vi "Set_Source.vi"(6 "Source Status":T7, 7 "Establish Exp Conditions":bool, 8 "Traverse line":T3 {"Carrier_2 Q (l/min)" format="%#.2f"; "Row Duration (mins)" format="%#.1f"; "Row No" min=0; "Trace Gas Concentration (%)" min=0.0 format="%#_4f"; "Carrier_1 Q (l/min)" format="%#.2f"; "Tunnel Speed" format="%#.2f"; "Start X" format="%#.2f"; "Start Y" format="%#.2f"; "Start Z" format="%#.2f"; "End X" format="%#.2f"; "End Y" format="%#.2f"; "End Z" format="%#.2f"; "Averaging time (min)" min=0.0 format="%#.2f"}, 9 "Simulate/Run":T6) -> (0 "Status Cluster":T1, 1 "Flowrates (kg/min)":dbl[](array[numeric]) format="%.2f", 2 "Time Source Started":dbl, 3 "Flowrates Achieved?":bool, 4 "Source requested?":bool, 5 "Source Est Time":dbl format="%.2f")   [LabVIEW 2016]
uses:
  ADAM Client/Sub VIs/ADAM Controls/Client_Source_Status.ctl
  Controls/User_Specific_mode.ctl
  Traverse_cluster.ctl
  Spacing.ctl
  Controls/Multi_run_mode.ctl
  Status_Cluster.ctl
  Multi_Run_Status.ctl
  Globals/Trav_pos_global.vi
  Globals/Extra_Commands_Global.vi
panel:
  # "X           Y            Z"
  # "Start"
  # "End"
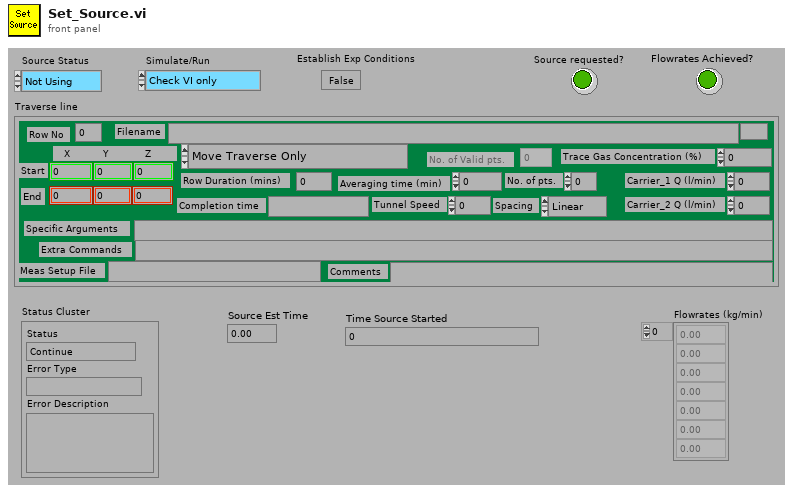
[diagram p1: front panel]
types:
  T1 = typedef "Status_Cluster.ctl" = cluster{"Status":T2, "Error Type":string, "Error Description":string}
  T2 = typedef "Multi_Run_Status.ctl" = enum16{"Continue", "Jump to Next Point", "Jump to Next Row", "Jump To Fall Back", "Terminate Run"}
  T3 = typedef "Traverse_cluster.ctl" = cluster{"Start X":sgl, "Start Y":sgl, "Start Z":sgl, "End X":sgl, "End Y":sgl, "End Z":sgl, "No. of pts.":i32, "Spacing":T4, "Filename":path, "Tunnel Speed":dbl, "Averaging time (min)":dbl, "Extra Commands":string, "Carrier_1 Q (l/min)":dbl, "Carrier_2 Q (l/min)":dbl, "Trace Gas Concentration (%)":dbl, "Specific Arguments":string, "Comments":string, "Row No":i32, "Row Type Selector":T5, "Completion time":string, "Row Duration (mins)":dbl, "No. of Valid pts.":i32, "Meas Setup File":string}
  T4 = typedef "Spacing.ctl" = enum16{"Linear", "Log", "Gauss", "Specified", "N/A"}
  T5 = typedef "Multi_run_mode.ctl" = enum16{"Move Traverse Only", "Set Tunnel Speed Only", "Set Source Only", "Set Measurement Conditions", "Single Measurement", "Vertical Profile", "Lateral Profile", "Longitudinal Profile", "Explore Volume", "Multi-Axis Profile", "Auto Calibrate", "Meas Fast FID Bkgnd", "Check Beam Power", "Scanning Valve Measurement", "Run VI Named:", "Set ADAM Ch", "Wait (minutes)", "Send Message", "Synchronize With:", "Fall Back to this Row", "Turn Off Row Repeating", "Blank Row", "Traverse 3D Volume"}
  T6 = typedef "User_Specific_mode.ctl" = enum16{"Check VI only", "Run VI"}
  T7 = typedef "Client_Source_Status.ctl" = enum16{"Not Using", "Using", "Must Have"}
  T8 = cluster{"Carrier_1 Q (l/min)":dbl, "Carrier_2 Q (l/min)":dbl, "Trace Gas Concentration (%)":dbl}
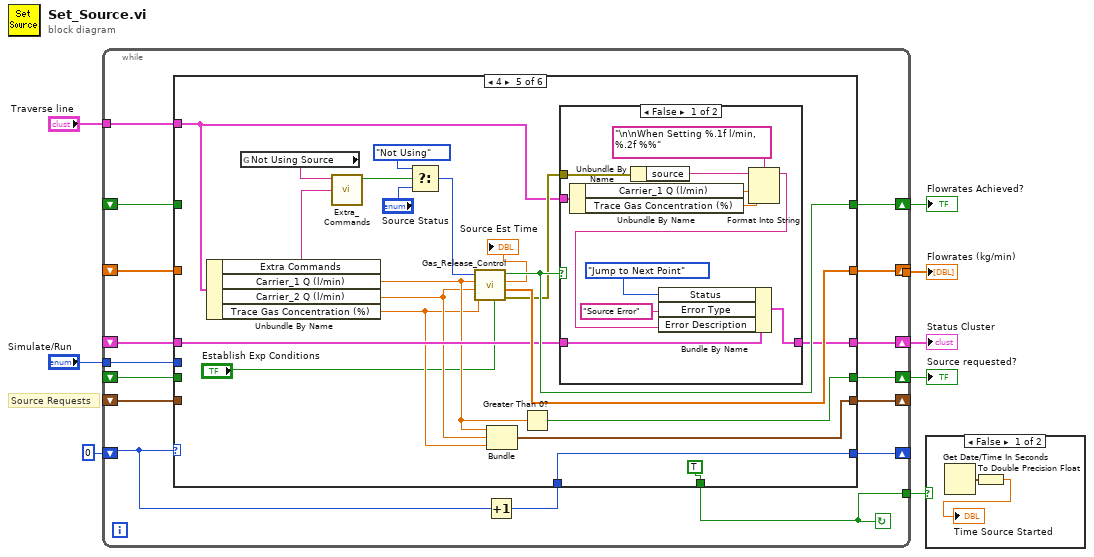
[diagram p0: block diagram]
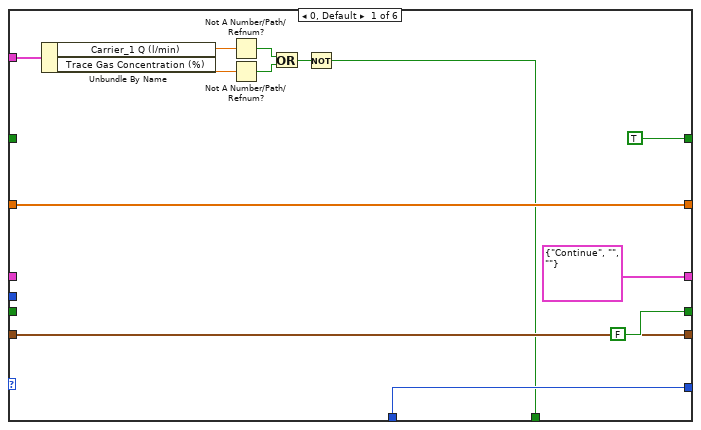
[diagram p3: hidden frame]
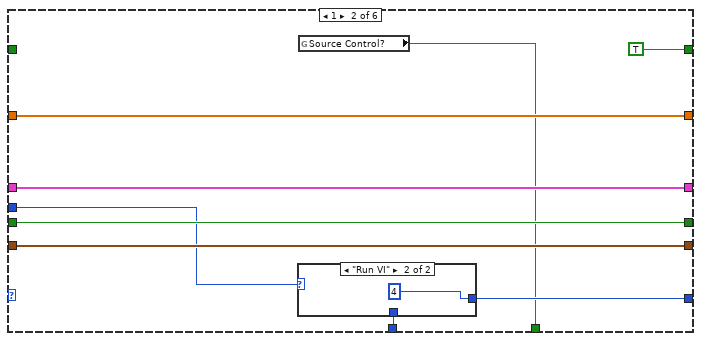
[diagram p4: hidden frame]
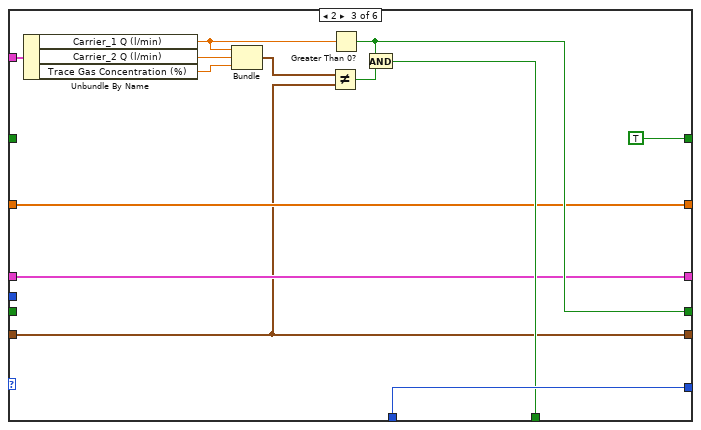
[diagram p6: hidden frame]
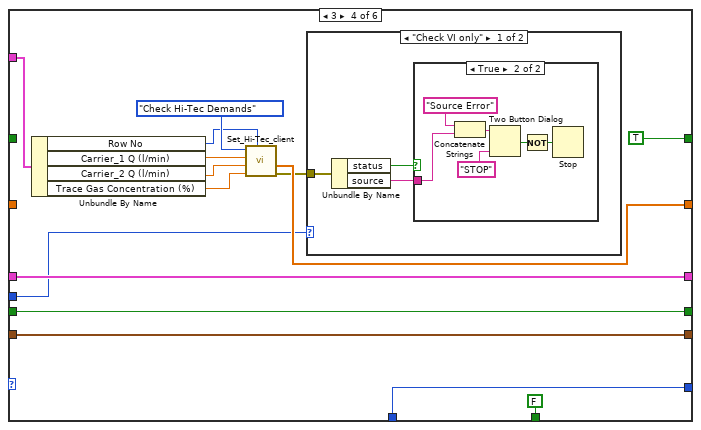
[diagram p7: hidden frame]
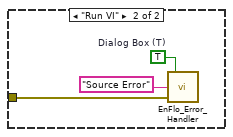
[diagram p9: hidden frame]
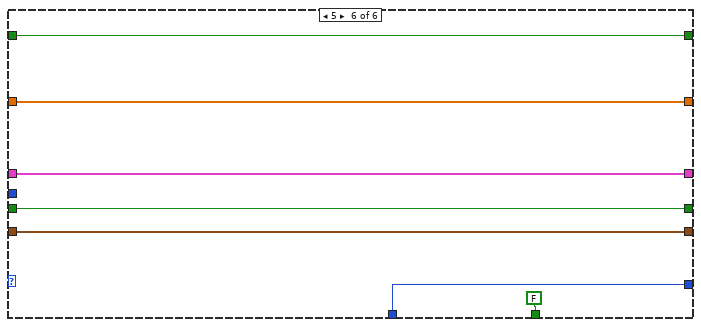
[diagram p11: hidden frame]
diagram:
  # "Source Requests"
  n1 = while {
    shift-left: _ -> [w12]
    shift-right: [w13] -> w4
    shift-left: _ -> [w14]
    shift-right: [w15] -> w5
    shift-left: _ -> [w16]
    shift-right: [w19] -> w6
    shift-left: 0 -> [w18]
    shift-right: [w20] -> _
    shift-left: _ -> [w21]
    shift-right: [w22] -> _
    tunnel: [w22] -> w8
    shift-left: _ -> [w24]
    shift-right: [w23] -> _
    tunnel: "Simulate/Run" -> [w11]
    tunnel: "Traverse line" -> [w10]
    tunnel: [w9] -> w1
    stop <- w9 continue-if-true
    n2 = Increment(x=w18) -> (x+1=w17:i32)
    n3 = case shown="4" w18 {
      tunnel: [w35 w46 w52 w71 w102 w123] -> w22
      tunnel: w24 -> [w32 w44 w50 w68 _ w127]
      tunnel: [w32 w44 w50 w68 w93 w127] -> w23
      tunnel: w21 -> [w35 w46 w52 _ _ w123]
      tunnel: [FALSE w40 w61 w69 w109 w128] -> w19
      tunnel: [TRUE ("Flowrates Achieved?") TRUE ("Flowrates Achieved?") TRUE ("Flowrates Achieved?") TRUE ("Flowrates Achieved?") w103 w122] -> w13
      tunnel: [w25 w38 w55 FALSE TRUE FALSE] -> w9
      tunnel: [w31 w43 w56 w67 w100 w126] -> w20
      tunnel: w17 -> [w31 w41 w56 w67 w100 w126]
      tunnel: w16 -> [_ w40 _ w69 _ w128]
      tunnel: [T1 {"Status"=enum."Continue", "Error Type"="", "Error Description"=""} ("Status Cluster") w42 w51 w65 w101 w124] -> w15
      tunnel: w14 -> [_ w42 w51 w65 w97 w124]
      tunnel: w12 -> [_ _ _ _ _ w122]
      tunnel: w11 -> [_ w39 _ w63 _ _]
      tunnel: w10 -> [w29 _ w49 w62 w91 _]
      frame 0, Default {
        n4 = Unbundle By Name(w29) -> ("Carrier_1 Q (l/min)"=w37:dbl, "Trace Gas Concentration (%)"=w30:dbl)
        n5 = Not A Number/Path/Refnum?(number/path/refnum=w37) -> (NaN/Path/Refnum?=w27:bool)
        n6 = Not A Number/Path/Refnum?(number/path/refnum=w30) -> (NaN/Path/Refnum?=w28:bool)
        n7 = Or(x=w27, y=w28) -> (x .or. y?=w26:bool)
        n8 = Not(x=w26) -> (.not. x?=w25:bool)
      }
      frame 1 {
        n9 = case shown="\"Run VI\"" w39 {
          tunnel: [w47 4] -> w43
          tunnel: w41 -> [w47 _]
          frame "Check VI only" {
          }
          frame "Run VI" {
          }
        }
        n10 = global read "Trav_pos_global.vi" "Source Control?"() -> (w38:bool)
      }
      frame 2 {
        n11 = Unbundle By Name(w49) -> ("Carrier_1 Q (l/min)"=w58:dbl, "Carrier_2 Q (l/min)"=w60:dbl, "Trace Gas Concentration (%)"=w59:dbl)
        n12 = Bundle("Carrier_1 Q (l/min)"=w58, "Carrier_2 Q (l/min)"=w60, "Trace Gas Concentration (%)"=w59) -> (w54:T8)  [unwired: 1 out]
        n13 = Not Equal?(x=w54, y=w50) -> (x != y?=w57:bool)
        n14 = Greater Than 0?(x=w58) -> (x > 0?=w61:bool)
        n15 = And(x=w61, y=w57) -> (x .and. y?=w55:bool)
      }
      frame 3 {
        n16 = Unbundle By Name(w62) -> ("Row No"=w72:i32, "Carrier_1 Q (l/min)"=w75:dbl, "Carrier_2 Q (l/min)"=w74:dbl, "Trace Gas Concentration (%)"=w73:dbl)
        n17 = call "Set_Hi-Tec_client.vi"("Row No"=w72, "Strength (% by volume)"=w73, "Carrier_2 Q (l/min)"=w74, "Carrier_1 Q (l/min)"=w75, "Mode"=enum16{"Control Hi-Tec", "Check Hi-Tec Demands"}."Check Hi-Tec Demands") -> ("error out"=w64:errorcluster, "Flowrates (kg/min)"=w71:dbl[])  [unwired: 3 out]
        n18 = case shown="\"Check VI only\"" w63 {
          tunnel: w64 -> [w79 w88]
          frame "Check VI only" {
            n19 = Unbundle By Name(w79) -> ("status"=w77:bool, "source"=w78:string)
            n20 = case shown="True" w77 {
              tunnel: w78 -> [_ w84]
              frame False {
              }
              frame True {
                n21 = Concatenate Strings("Source Error" ("Error Type"), w84) -> (w83:string)
                n22 = Two Button Dialog(message=w83, 1:"STOP" ("F button name (\"Cancel\")")) -> (T button?=w81:bool)  [unwired: 1 out]
                n23 = Not(x=w81) -> (.not. x?=w80:bool)
                n24 = Stop(stop? (T)=w80) -> ()
              }
            }
          }
          frame "Run VI" {
            w86 = TRUE  # Dialog Box (T)
            n25 = call "EnFlo_Error_Handler.vi"("error in (no error)"=w88, "Error Type"="Source Error", "Dialog Box (T)"=w86) -> ()  [unwired: 3 out]
          }
        }
      }
      frame 4 {
        n26 = Unbundle By Name(w91) -> ("Extra Commands"=w89:string, "Carrier_1 Q (l/min)"=w96:dbl, "Carrier_2 Q (l/min)"=w95:dbl, "Trace Gas Concentration (%)"=w94:dbl)
        n27 = global read "Extra_Commands_Global.vi" "Not Using Source"() -> (w106:string)
        n28 = call "Extra_Commands.vi"("String to Search"=w89, "Command"=w106) -> ("Command Found"=w105:bool)  [unwired: 1 in, 4 out]
        n29 = Select(t=Client_Source_Status."Not Using" ("Source Status"), s=w105, f="Source Status") -> (s? t:f=w104:T7)
        n30 = call "Gas_Release_Control.vi"("Establish Exp Conditions"="Establish Exp Conditions", "Strength (% by volume)"=w94, "Carrier_2 Q (l/min)"=w95, "Carrier_1 Q (l/min)"=w96, "Source Status"=w104) -> ("error out"=w92:errorcluster, "Flowrates (kg/min)"=w102:dbl[], "Source Est Time (s)"=→"Source Est Time":dbl, "Flowrates Achieved?"=w103:bool)  [unwired: 1 in]
        n31 = Bundle("Carrier_1 Q (l/min)"=w96, "Carrier_2 Q (l/min)"=w95, "Trace Gas Concentration (%)"=w94) -> (w93:T8)  [unwired: 1 out]
        n32 = Greater Than 0?(x=w96) -> (x > 0?=w109:bool)
        n33 = case shown="False" w103 {
          tunnel: [w116 w121] -> w101
          tunnel: w97 -> [w117 w121]
          tunnel: w91 -> [w112 _]
          tunnel: w92 -> [w111 _]
          frame False {
            n34 = Unbundle By Name(w112) -> ("Carrier_1 Q (l/min)"=w119:dbl, "Trace Gas Concentration (%)"=w118:dbl)
            n35 = Unbundle By Name(w111) -> ("source"=w110:string)
            n36 = Format Into String(format string="\n\nWhen Setting %.1f l/min, %.2f %%" ("Format String"), initial string=w110, w119, w118) -> (resulting string=w113:string)  [unwired: 1 in, 1 out]
            n37 = Bundle By Name(cluster=w117, "Status"=Multi_Run_Status."Jump to Next Point", "Error Type"="Source Error" ("Bundle Element"), "Error Description"=w113) -> (w116:T1)
          }
          frame True {
          }
        }
      }
      frame 5 {
      }
    }
  }
  "Flowrates (kg/min)" <- w8
  "Source requested?" <- w6
  "Flowrates Achieved?" <- w4
  "Status Cluster" <- w5
  n38 = case shown="False" w1 {
    frame False {
      n39 = Get Date/Time In Seconds() -> (seconds since 1Jan1904=w130:timestamp)
      n40 = To Double Precision Float(number=w130) -> (double precision float=→"Time Source Started":dbl)
    }
    frame True {
    }
  }
